vi "Recover_last_framescan_on_linescan_display.vi"(8 "error in (no error)":errorcluster, 10 "Time stamp of last confirm":string, 11 "Last framescan image (updates when pressing \"Confirm\")":i16[][](array[numeric])) -> (0 "error out":errorcluster)   [LabVIEW 2012]
uses:
  GFG/GFGImageRefsGet.vi
  GFG/GFG library.lvlib
  <vilib>/vision/NI_Vision_Development_Module.lvlib
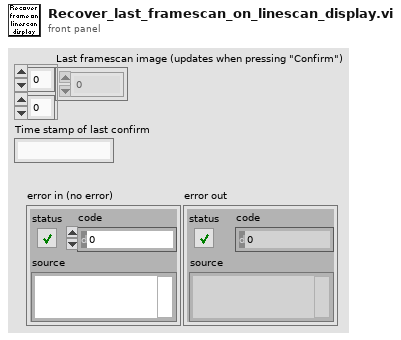
[diagram p1: front panel]
types:
  T1 = cluster{"Desired Font (Application)":enum16{"User-specified Font", "Application Font", "System Font", "Dialog Font"}, "[User-specified Font]":cluster{"Font Name":string, "Size":i16, "Strikeout?":bool, "Italic?":bool, "Underline?":bool, "Outline?":bool, "Shadow?":bool, "Bold?":bool, "Rotation Angle":dbl}, "Horizontal Alignment":i16, "Vertical Alignment":i16}
  T2 = typedef "ROI Descriptor" = cluster{"Global Rectangle":i32[], "Contours":cluster{"ID":enum32{"External", "Internal"}, "Type":u32, "Coordinates":i32[]}[]}
  T3 = cluster{"Left":i32, "Top":i32, "Right":i32, "Bottom":i32}
  T4 = typedef "IMAQ Image.ctl" = refnum<image>
  T5 = cluster{"Channel 1 small":T4, "Channel 2 small":T4, "Channel 3 small":T4, "Channel 4 small":T4, "Channel 1 large":T4, "Channel 2 large":T4, "Channel 3 large":T4, "Channel 4 large":T4, "RGB overlay":T4, "ROI Image display":T4, "arb line scan display":T4, "Channel 5 large":T4}
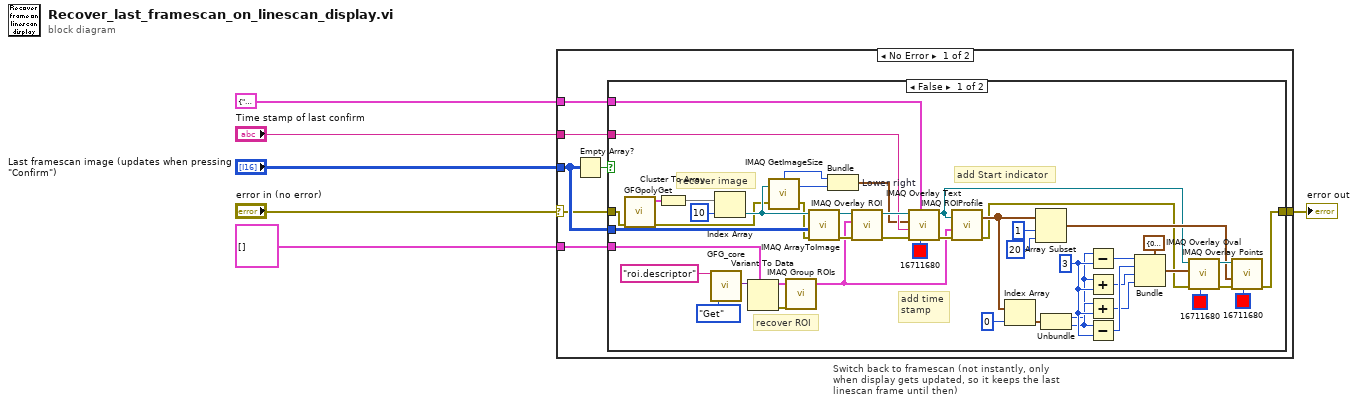
[diagram p0: block diagram]
diagram:
  n1 = case shown="No Error" "error in (no error)" {
    selector: "error in (no error)" -> [w8 w63]
    tunnel: "Last framescan image (updates when pressing \"Confirm\")" -> [w13 _]
    tunnel: "Time stamp of last confirm" -> [w12 _]
    tunnel: T2[] [] ("ROI Descriptors out") -> [w11 _]
    tunnel: T1 {"Desired Font (Application)"=enum."Application Font", "[User-specified Font]"={"Font Name"="", "Size"=15, "Strikeout?"=FALSE, "Italic?"=FALSE, "Underline?"=FALSE, "Outline?"=FALSE, "Shadow?"=FALSE, "Bold?"=TRUE, "Rotation Angle"=0.0}, "Horizontal Alignment"=2, "Vertical Alignment"=0} ("Font, Size & Style") -> [w9 _]
    tunnel: [w7 w63] -> w1
    frame No Error {
      n2 = Empty Array?(array=w13) -> (empty?=w10:bool)
      n3 = case "Switch back to framescan (not instantly, only when display gets updated, so it keeps the last linescan frame until then)" shown="False" w10 {
        tunnel: w13 -> [w58 _]
        tunnel: w11 -> [w54 _]
        tunnel: w12 -> [w48 _]
        tunnel: w9 -> [w24 _]
        tunnel: w8 -> [w16 w62]
        tunnel: [w15 w62] -> w7
        frame False {
          w42 = 3 ("y")
          # "add Start indicator"
          # "recover image"
          # "recover ROI"
          # "add time\nstamp"
          n4 = call-poly "GFGpolyGet.vi"("error in (no error)"=w16) -> ("error out"=w18:errorcluster, "Image Refs Out"=w61:T5)  [unwired: 9 in]
          n5 = Cluster To Array(cluster=w61) -> (array=w59:T4[])
          n6 = call "GFG_core.vi"("Variable Name in"="roi.descriptor", "Action"=enum16{"Init", "Set", "Get"}."Get") -> ("Variant Out"=w57:variant)  [unwired: 11 in, 6 out]
          n7 = Index Array(array=w59, index=10) -> (element=w44:T4)
          n8 = Variant To Data(type=w54, Variant=w57) -> (data=w52:T2[], error out=w51:errorcluster)  [unwired: 1 in]
          n9 = call "IMAQ GetImageSize"("Image"=w44, "error in (no error)"=w18) -> ("Y Resolution"=w45:i32, "X Resolution"=w46:i32, "error out"=w17:errorcluster)  [unwired: 2 in]
          n10 = call "IMAQ Group ROIs"("error in (no error)"=w51, "ROI Descriptors"=w52) -> ("ROI Descriptor out"=w14:T2)  [unwired: 2 in, 1 out]
          n11 = call "IMAQ ArrayToImage"("error in (no error)"=w17, "Image Pixels (I16)"=w58, "Image"=w44) -> ("error out"=w19:errorcluster, "Image Out"=w53:T4)  [unwired: 7 in]
          n12 = Bundle "Lower right"("X Resolution"=w46, "Y Resolution"=w45) -> (w43:cluster{"X Resolution":i32, "Y Resolution":i32})  [unwired: 1 in]
          n13 = call "IMAQ Overlay ROI"("error in (no error)"=w19, "ROI Descriptor"=w14, "Image"=w53) -> ("error out"=w49:errorcluster, "Image Out"=w50:T4)  [unwired: 7 in]
          n14 = call "IMAQ Overlay Text"("Text Color (black)"=u32 16711680, "Font, Size & Style"=w24, "error in (no error)"=w49, "String"=w48, "Origin"=w43, "Image"=w50) -> ("error out"=w23:errorcluster, "Image Out"=w22:T4)  [unwired: 4 in]
          n15 = call "IMAQ ROIProfile"("error in (no error)"=w23, "ROI Descriptor"=w14, "Image"=w22) -> ("error out"=w20:errorcluster, "Pixel Coordinates"=w36:cluster{"X":u32, "Y":u32}[])  [unwired: 1 in, 3 out]
          n16 = Index Array(array=w36, index=0) -> (element=w27:cluster{"X":u32, "Y":u32})
          n17 = Array Subset(array=w36, index=1, length=20) -> (w39:cluster{"X":u32, "Y":u32}[])
          n18 = Unbundle(w27) -> ("X"=w33:u32, "Y"=w34:u32)
          n19 = Subtract(x=w33, y=w42) -> (x-y=w29:u32)
          n20 = Add(x=w33, y=w42) -> (x+y=w28:u32)
          n21 = Add(x=w34, y=w42) -> (x+y=w30:u32)
          n22 = Subtract(x=w34, y=w42) -> (x-y=w31:u32)
          n23 = Bundle(cluster=T3 {"Left"=0, "Top"=0, "Right"=0, "Bottom"=0} ("Bounding Rectangle"), "Left"=w29, "Top"=w31, "Right"=w28, "Bottom"=w30) -> (w35:T3)
          n24 = call "IMAQ Overlay Oval"("Color"=u32 16711680, "error in (no error)"=w20, "Bounding Rectangle"=w35, "Image"=w22) -> ("error out"=w21:errorcluster, "Image Out"=w41:T4)  [unwired: 6 in]
          n25 = call "IMAQ Overlay Points"("Color"=u32 16711680, "error in (no error)"=w21, "Array of Points"=w39, "Image"=w41) -> ("error out"=w15:errorcluster)  [unwired: 6 in, 1 out]
        }
        frame True {
        }
      }
    }
    frame Error {
    }
  }
  "error out" <- w1
